vi "G4BaseTemplate_Simple_5x6x5_ReadWriteAttribute.vi"(0 "reference in":refnum<class "G4BaseTemplate_Simple_5x6x5.lvclass">, 11 "error in (no error)":errorcluster) -> (4 "reference out":refnum<class "G4BaseTemplate_Simple_5x6x5.lvclass">, 15 "error out":errorcluster)   [LabVIEW 2014]
uses:
  <resource>/Framework/Providers/Open_GDS/ClassProviders/Provider_EndevoGOOP400/Templates/G4BaseTemplate_Simple_5x6x5/G4BaseTemplate_Simple_5x6x5.lvclass
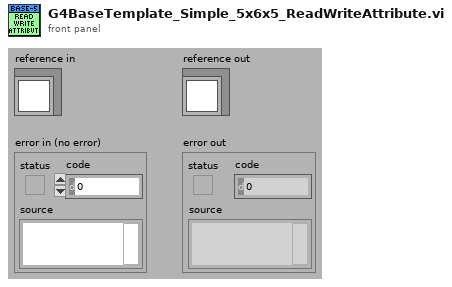
[diagram p1: front panel]
types:
  T1 = typedef "G4BaseTemplate_Simple_5x6x5.lvclass/ObjectAttributes.ctl" = cluster{"Attribute1":dbl}
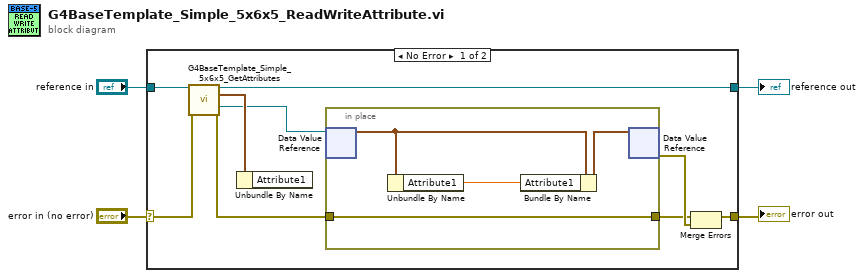
[diagram p0: block diagram]
diagram:
  n1 = case shown="No Error" "error in (no error)" {
    selector: "error in (no error)" -> [w12 w19]
    tunnel: [w8 w19] -> w3
    tunnel: [w9 w18] -> w1
    tunnel: "reference in" -> [w13 w18]
    frame No Error {
      n2 = call <resource>:"G4BaseTemplate_Simple_5x6x5_GetAttributes.vi"("reference in"=w13, "error in (no error)"=w12) -> ("reference out"=w9:refnum<class "G4BaseTemplate_Simple_5x6x5.lvclass">, "Data"=w11:T1, "DataRef"=w7:refnum<data-value>, "error out"=w6:errorcluster)  [unwired: 10 in]
      n3 = Unbundle By Name(w11) -> ()  [unwired: 1 out]
      n4 = in-place {
        in-place-border: w6 -> [w16]
        in-place-border: [w16] -> w5
        n5 = in-place-dvr #1(w7) -> (w15:T1)  [unwired: 1 out]
        n6 = Unbundle By Name(w15) -> ("Attribute1"=w14:dbl)
        n7 = Bundle By Name(cluster=w15, "Attribute1"=w14) -> (w17:T1)
        n8 = in-place-dvr #1(w17) -> (w10:errorcluster)  [unwired: 1 out]
      }
      n9 = Merge Errors(w5, w10) -> (w8:errorcluster)
    }
    frame Error {
    }
  }
  "error out" <- w3
  "reference out" <- w1
